vi "clear Session Data.vi"(0 "Session in":refnum<class "Test Number and Bin Generator.lvclass">=refnum, 11 "error in":errorcluster) -> (4 "Session out":refnum<class "Test Number and Bin Generator.lvclass">, 15 "error out":errorcluster)   [LabVIEW 2018, in "Test Number and Bin Generator.lvlib" / "Test Number and Bin Generator.lvclass"]
uses:
  Test Number and Bin Generator.lvclass
  Test Number and Bin Generator.lvclass/Test Number and Bin Generator.ctl
  Typedefs/Evaluation QMH.ctl
  Plugins/TestStand API Tools (TSAT).lvlibp/Evaluation Actions/Includes/Controls/TSAT Eval SI Unit Scaling.ctl
  Plugins/TestStand API Tools (TSAT).lvlibp/Evaluation Actions/Includes/Controls/TSAT Evaluation Type.ctl
  Plugins/Sequence Automation Session.lvlibp/Sequence Automation Session.lvclass
  Plugins/TestStand API Tools (TSAT).lvlibp/Evaluation Actions/TSAT Evaluation Actions.lvlib
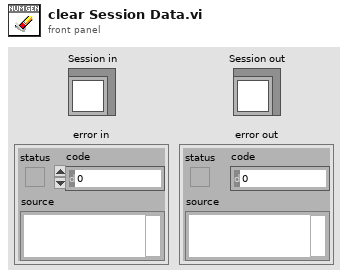
[diagram p1: front panel]
types:
  T1 = typedef "Test Number and Bin Generator.lvlib/Test Number and Bin Generator.lvclass/Evaluation QMH.ctl" = cluster{"Command":string, "Evaluations":cluster{"Test Name":string, "Pin":string, "Units":string, "SI Scaling":T2, "Test Number":i32, "Published Data Id":string, "Low Limit":dbl, "High Limit":dbl, "Export Data Location":string, "Software Bin":i64, "Evaluation Type":T3, "Test Data Source":string}[]}
  T2 = typedef "TestStand API Tools (TSAT).lvlibp/TSAT Evaluation Actions.lvlib/TSAT Eval SI Unit Scaling.ctl" = i16
  T3 = typedef "TestStand API Tools (TSAT).lvlibp/TSAT Evaluation Actions.lvlib/TSAT Evaluation Type.ctl" = enum16{"Numeric Limit", "Pass/Fail", "None"}
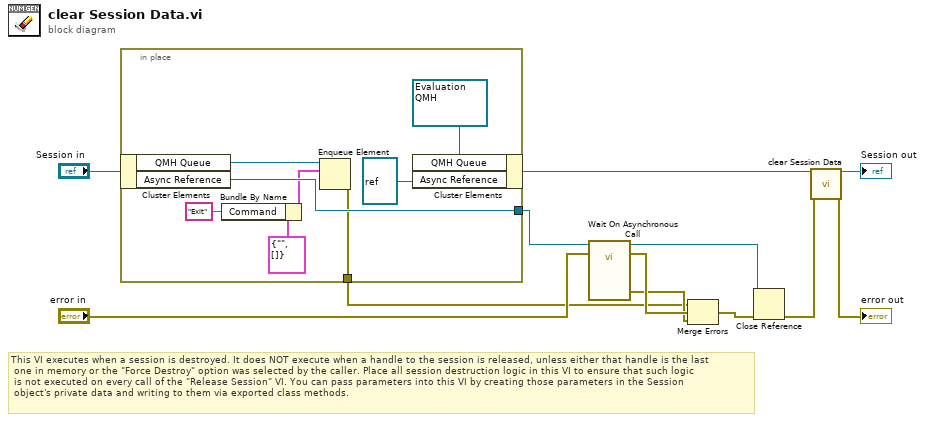
[diagram p0: block diagram]
diagram:
  # "This VI executes when a session is destroyed. It does NOT execute when a handle to the session is released, unless either that handle is the last\n one in memory or the \"Force Destroy\" option was selected by the caller. Place all session destruction logic in this VI to ensure that such logic\n is not executed on every call of the \"Release Session\" VI. You can pass parameters into this VI by creating those parameters in the Session \n object's private data and writing to them via exported class methods."
  n1 = in-place {
    in-place-border: [w20] -> w10
    in-place-border: [w15] -> w1
    n2 = in-place-cluster #1("Session in") -> ("QMH Queue"=w19:refnum<queue>, "Async Reference"=w20:refnum<vi>)
    n3 = Bundle By Name(cluster=T1 {"Command"="", "Evaluations"=[]} ("element"), "Command"="Exit") -> (w16:T1)
    n4 = Enqueue Element(queue=w19, element=w16) -> (error out=w15:errorcluster)  [unwired: 2 in, 2 out]
    n5 = in-place-cluster #1("QMH Queue"=refnum<queue> refnum, "Async Reference"=refnum<vi> refnum) -> (w2:refnum<class "Test Number and Bin Generator.lvclass">)
  }
  n6 = call-by-ref "Wait On Asynchronous Call"(reference=w10, error in="error in") -> (reference out=w6:refnum<vi>, error out=w5:errorcluster, 0:"error out"=w4:errorcluster)  [unwired: 11 in]
  n7 = Merge Errors(w1, w5, w4) -> (w8:errorcluster)
  n8 = Close Reference(reference=w6, error in (no error)=w8) -> (error out=w7:errorcluster)
  n9 = call-parent "clear Session Data.vi"("OBJ - Measurement Session in"=w2, "error in"=w7) -> ("OBJ - Measurement Session out"=→"Session out":refnum<class "Test Number and Bin Generator.lvclass">, "error out"=→"error out":errorcluster)  [unwired: 12 in]
